vi "Start Build.vi"(0 "Open Directory?":bool, 1 "Build Packge?":bool, 2 "Progres Bar":refnum<vi>, 5 "Feed":T2(ring), 7 "Feed Path":path, 9 "Selected Measurements":T1[](array[typedef]), 11 "error in (no error)":errorcluster, 12 "Package Spec":string[][](array[string])) -> (4 "Status":string[](array[string]), 15 "error out":errorcluster)   [LabVIEW 2021, in "Packager Helpers.lvlib"]
uses:
  Packager Helpers.lvlib
  controls/Build Spec Details.ctl
  <vilib>/AppBuilder/AB_API_Simple/Set Build Specification Version (path).vi
  <vilib>/AppBuilder/AB_API_Simple/Build (path).vi
  Dictionary/Dictionary.lvlib
  <vilib>/AppBuilder/AB_API_Simple/NI_App_Builder_API.lvlib
  Path Functions/Path Functions.lvlib
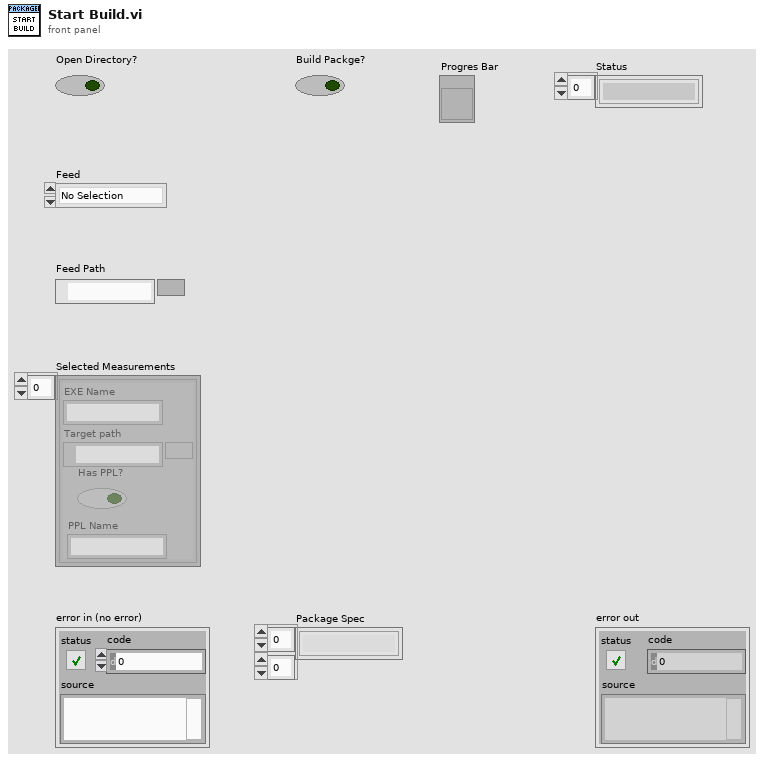
[diagram p1: front panel]
types:
  T1 = typedef "Packager Helpers.lvlib/Build Spec Details.ctl" = cluster{"EXE Name":string, "Target path":path, "Has PPL?":bool, "PPL Name":string}
  T2 = enum32{"No Selection", "CreateFeed", "AddtoFeed"}
  T3 = typedef "NI_App_Builder_API.lvlib/Build Specification Version.ctl" = cluster{"Major":u16, "Minor":u16, "Fix":u16, "Build":u16}
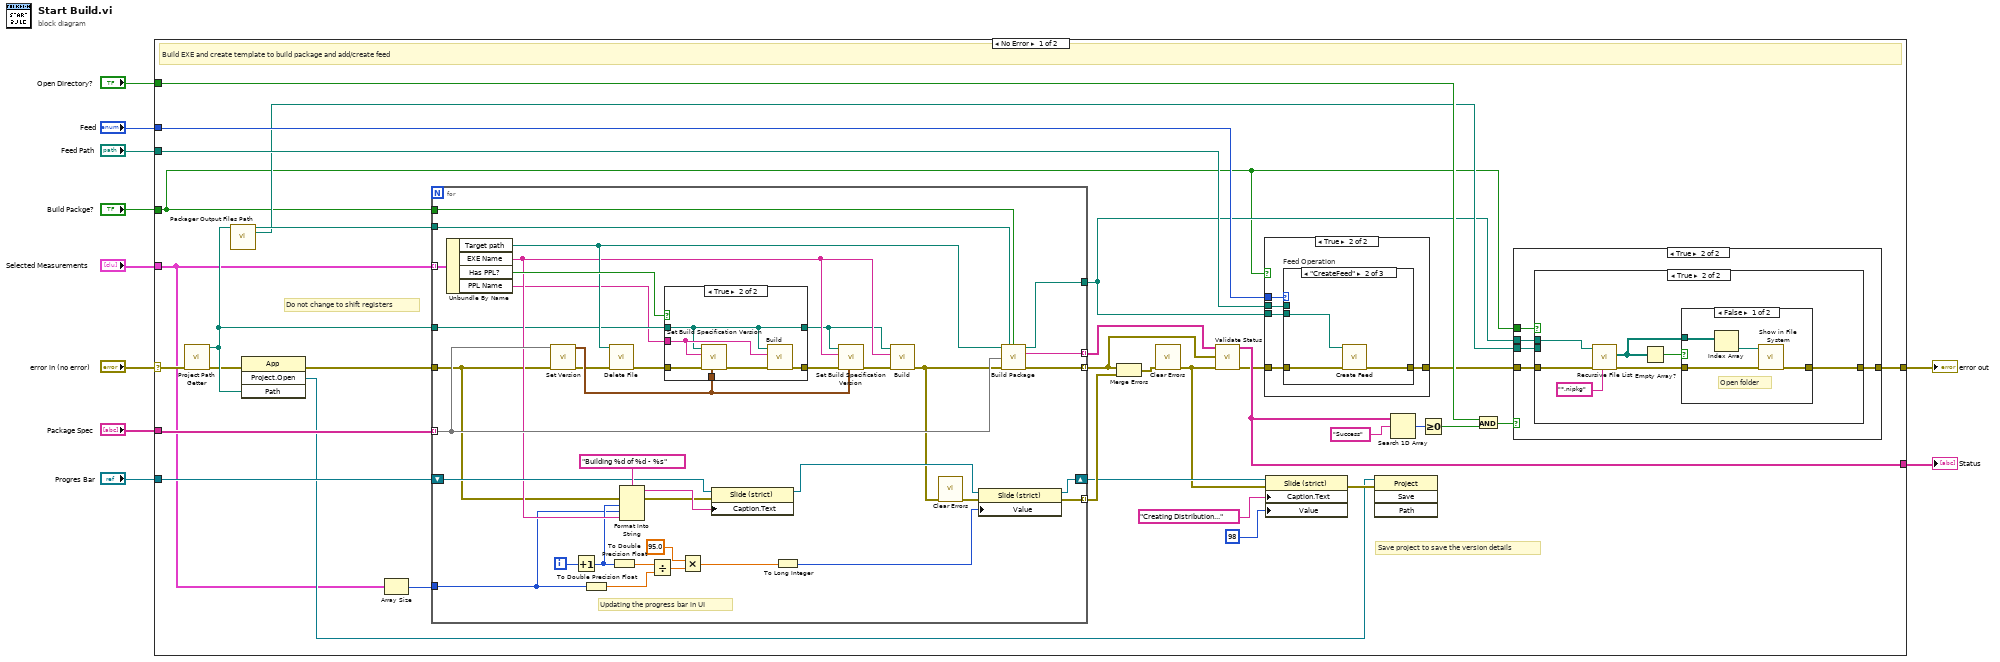
[diagram p0: block diagram]
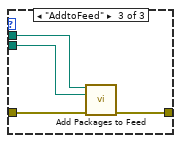
[diagram p4: hidden frame]
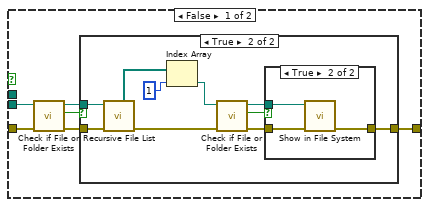
[diagram p7: hidden frame]
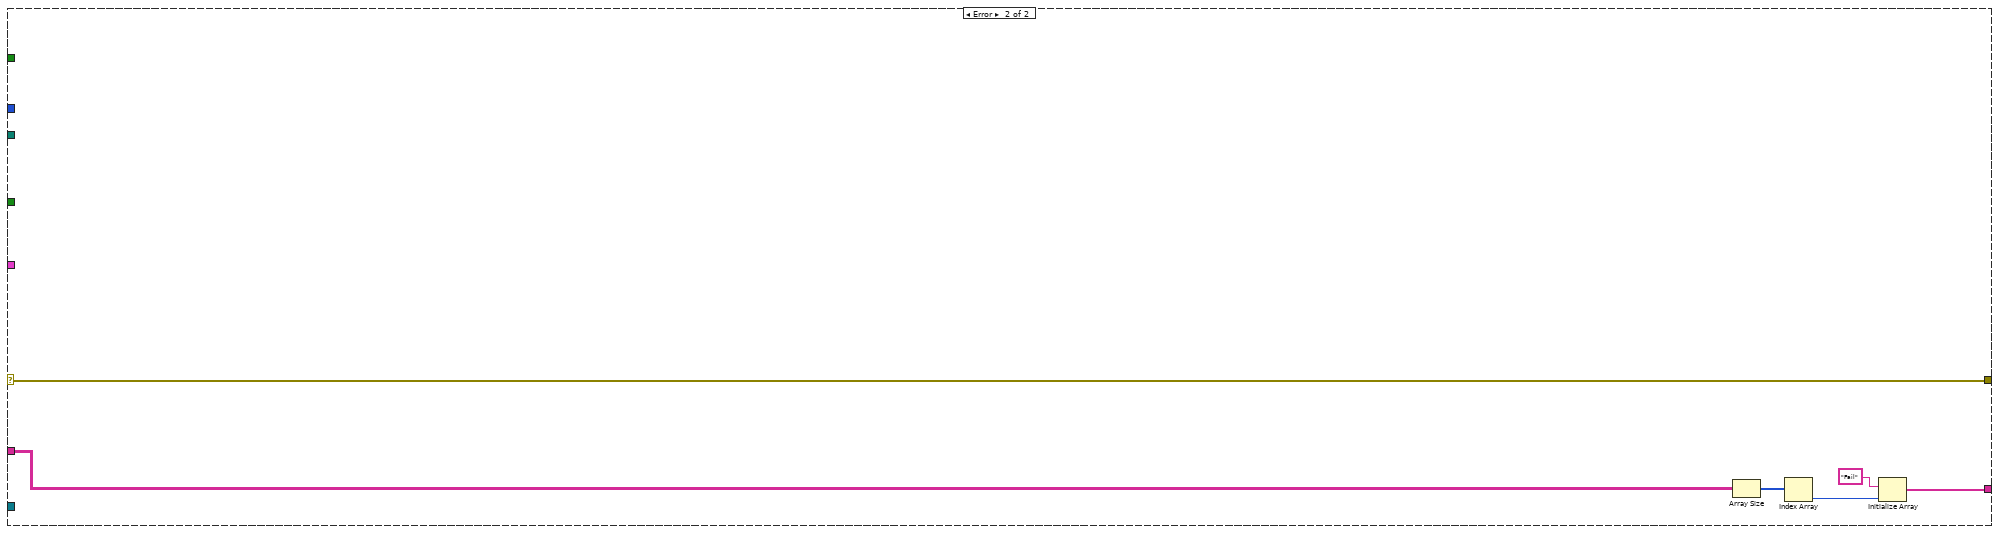
[diagram p11: hidden frame]
diagram:
  n1 = case shown="No Error" "error in (no error)" {
    selector: "error in (no error)" -> [w29 w142]
    tunnel: "Package Spec" -> [w43 w147]
    tunnel: [w37 w144] -> w9
    tunnel: "Progres Bar" -> [w27 _]
    tunnel: "Open Directory?" -> [w33 _]
    tunnel: "Feed" -> [w39 _]
    tunnel: "Feed Path" -> [w38 _]
    tunnel: "Build Packge?" -> [w13 _]
    tunnel: "Selected Measurements" -> [w20 _]
    tunnel: [w14 w142] -> w10
    frame No Error {
      # "Do not change to shift registers"
      # "Save project to save the version details"
      # "Build EXE and create template to build package and add/create feed"
      n2 = call "Project Path Getter.vi"("error in (no error)"=w29) -> ("Path"=w31:path, "error out"=w28:errorcluster)  [unwired: 13 in]
      n3 = call "Packager Output Files Path.vi"("Project Path"=w31) -> ("Package Path"=w32:path, "Build Outputs Path"=w30:path)  [unwired: 13 in]
      n4 = invoke class="App" method="Project.Open"(error in=w28, "Path"=w31) -> (error out=w11:errorcluster, "Project:Open"=w21:refnum<vi>)  [unwired: 2 in, 2 out]
      n5 = Array Size(array=w20) -> (size(s)=w41:i32)
      n6 = for {
        tunnel: w11 -> [w69]
        tunnel: w20 -> [w94] mode=indexing
        tunnel: w13 -> [w84]
        tunnel: w43 -> [w77] mode=indexing
        tunnel: [w93] -> w17
        tunnel: [w62] -> w25 mode=indexing
        tunnel: [w92] -> w42 mode=indexing
        tunnel: w41 -> [w59]
        tunnel: [w81] -> w40 mode=indexing
        shift-right: [w79] -> w24
        shift-left: w27 -> [w90]
        tunnel: w31 -> [w72]
        tunnel: w32 -> [w75]
        i -> [w58]
        # "Updating the progress bar in UI"
        n7 = Unbundle By Name(w94) -> ("Target path"=w76:path, "EXE Name"=w73:string, "Has PPL?"=w78:bool, "PPL Name"=w71:string)
        n8 = call "Set Version.vi"("Package Spec"=w77, "error in (no error)"=w69) -> ("Build Specification Version"=w70:T3, "error out"=w68:errorcluster)  [unwired: 12 in]
        n9 = Increment(x=w58) -> (x+1=w60:i32)
        n10 = To Double Precision Float(number=w59) -> (double precision float=w83:dbl)
        n11 = call "Delete File.vi"("File or Folder Path"=w76, "error in (no error)"=w68) -> ("error out"=w67:errorcluster)  [unwired: 13 in]
        n12 = To Double Precision Float(number=w60) -> (double precision float=w85:dbl)
        n13 = Format Into String(format string="Building %d of %d - %s", error in=w69, w60, w59, w73) -> (resulting string=w89:string, error out=w61:errorcluster)  [unwired: 1 in]
        n14 = Divide(x=w85, y=w83) -> (x/y=w88:dbl)
        n15 = case shown="True" w78 {
          tunnel: w72 -> [w95 w97]
          tunnel: w70 -> [_ w102]
          tunnel: w71 -> [_ w101]
          tunnel: w67 -> [w96 w100]
          tunnel: [w96 w98] -> w66
          tunnel: [w95 w97] -> w65
          frame False {
          }
          frame True {
            n16 = call-poly <vilib>:"Set Build Specification Version.vi"("Build Specification Version"=w102, "error in (no error)"=w100, "Name of build specification"=w101, "Path to project"=w97) -> ("error out"=w99:errorcluster)  [unwired: 7 in]
            n17 = call-poly <vilib>:"Build.vi"("error in (no error)"=w99, "Name of build specification (if empty: build all)"=w101, "Path to project"=w97) -> ("error out"=w98:errorcluster)  [unwired: 7 in, 1 out]
          }
        }
        n18 = Multiply(x=95.0 ("y"), y=w88) -> (x*y=w86:dbl)
        n19 = property class="Slide (strict)"(reference=w90, error in=w61, "Caption.Text"=w89) -> (reference out=w74:refnum<vi>)  [unwired: 1 out]
        n20 = To Long Integer(number=w86) -> (32bit integer=w80:i32)
        n21 = call-poly <vilib>:"Set Build Specification Version.vi"("Build Specification Version"=w70, "error in (no error)"=w66, "Name of build specification"=w73, "Path to project"=w65) -> ("error out"=w64:errorcluster)  [unwired: 7 in]
        n22 = call-poly <vilib>:"Build.vi"("error in (no error)"=w64, "Name of build specification (if empty: build all)"=w73, "Path to project"=w65) -> ("error out"=w63:errorcluster)  [unwired: 7 in, 1 out]
        n23 = call <vilib>:"Clear Errors.vi"("error in (no error)"=w63) -> ("error out"=w82:errorcluster)  [unwired: 5 in, 1 out]
        n24 = property class="Slide (strict)"(reference=w74, error in=w82, "Value"=w80) -> (reference out=w79:refnum<vi>, error out=w81:errorcluster)
        n25 = call "Build Package.vi"("Destination Path"=w76, "Package Path"=w75, "Build Package?"=w84, "Package Spec"=w77, "error in (no error)"=w63) -> ("Package Directory"=w93:path, "Error Message"=w92:string, "error out"=w62:errorcluster)  [unwired: 8 in]
      }
      n26 = Merge Errors(w25, w40) -> (w26:errorcluster)
      n27 = call <vilib>:"Clear Errors.vi"("error in (no error)"=w26) -> ("error out"=w23:errorcluster)  [unwired: 5 in, 1 out]
      n28 = call "Validate Status.vi"("Error Msg[]"=w42, "Error[]"=w25, "error in (no error)"=w23) -> ("Status"=w37:string[], "error out"=w16:errorcluster)  [unwired: 11 in]
      n29 = case shown="True" w13 {
        tunnel: w39 -> [_ w49]
        tunnel: w38 -> [_ w48]
        tunnel: w17 -> [_ w47]
        tunnel: w16 -> [w44 w46]
        tunnel: [w44 w45] -> w15
        frame False {
        }
        frame True {
          n30 = case "Feed Operation" shown="\"CreateFeed\"" w49 {
            tunnel: w48 -> [_ _ w57]
            tunnel: w47 -> [_ w53 w56]
            tunnel: w46 -> [w50 w52 w55]
            tunnel: [w50 w51 w54] -> w45
            frame "No Selection" {
            }
            frame "CreateFeed" {
              n31 = call "Create Feed.vi"("Packages Path"=w53, "error in (no error)"=w52) -> ("error out"=w51:errorcluster)  [unwired: 13 in]
            }
            frame "AddtoFeed" {
              n32 = call "Add Packages to Feed.vi"("Feed Path"=w57, "Packages Path"=w56, "error in (no error)"=w55) -> ("error out"=w54:errorcluster)  [unwired: 12 in]
            }
          }
        }
      }
      n33 = property class="Slide (strict)"(reference=w24, error in=w23, "Caption.Text"="Creating Distribution...", "Value"=98) -> (error out=w22:errorcluster)  [unwired: 1 out]
      n34 = invoke class="Project" method="Save"(reference=w21, error in=w22) -> ()  [unwired: 2 in, 4 out]
      n35 = Search 1D Array(1D array=w37, element="Success") -> (index of element=w35:i32)  [unwired: 1 in]
      n36 = Greater Or Equal To 0?(x=w35) -> (x >= 0?=w34:bool)
      n37 = And(x=w33, y=w34) -> (x .and. y?=w12:bool)
      n38 = case shown="True" w12 {
        tunnel: w17 -> [_ w108]
        tunnel: w30 -> [_ w107]
        tunnel: [w103 w105] -> w14
        tunnel: w15 -> [w103 w106]
        tunnel: w13 -> [_ w104]
        frame False {
        }
        frame True {
          n39 = case shown="True" w104 {
            tunnel: w108 -> [_ w136]
            tunnel: w107 -> [w113 _]
            tunnel: w106 -> [w112 w135]
            tunnel: [w110 w131] -> w105
            frame False {
              n40 = call <vilib>:"Check if File or Folder Exists.vi"("error in (no error)"=w112, "path"=w113) -> ("error out"=w111:errorcluster, "file or folder exists?"=w114:bool, "dup path"=w109:path)  [unwired: 7 in]
              n41 = case shown="True" w114 {
                tunnel: w111 -> [w115 w122]
                tunnel: [w115 w117] -> w110
                tunnel: w109 -> [_ w116]
                frame False {
                }
                frame True {
                  n42 = call <vilib>:"Recursive File List.vi"("error in (no error)"=w122, "Folder Path"=w116) -> ("error out"=w120:errorcluster, "All Folders"=w125:path[])  [unwired: 5 in, 3 out]
                  n43 = Index Array(array=w125, index=1) -> (element=w124:path)
                  n44 = call <vilib>:"Check if File or Folder Exists.vi"("error in (no error)"=w120, "path"=w124) -> ("error out"=w123:errorcluster, "file or folder exists?"=w119:bool, "dup path"=w118:path)  [unwired: 7 in]
                  n45 = case shown="True" w119 {
                    tunnel: w123 -> [w126 w128]
                    tunnel: w118 -> [_ w129]
                    tunnel: [w126 w127] -> w117
                    frame False {
                    }
                    frame True {
                      n46 = call <vilib>:"Show in File System.vi"("error in (no error)"=w128, "file or directory path"=w129) -> ("error out"=w127:errorcluster)  [unwired: 9 in]
                    }
                  }
                }
              }
            }
            frame True {
              n47 = call <vilib>:"Recursive File List.vi"("pattern"="*.nipkg", "error in (no error)"=w135, "Folder Path"=w136) -> ("error out"=w132:errorcluster, "All Files in Dir"=w134:path[])  [unwired: 4 in, 3 out]
              n48 = Empty Array?(array=w134) -> (empty?=w133:bool)
              n49 = case shown="False" w133 {
                tunnel: w132 -> [w138 w141]
                tunnel: w134 -> [w140 _]
                tunnel: [w137 w141] -> w131
                frame False {
                  # "Open folder"
                  n50 = Index Array(array=w140) -> (element=w139:path)  [unwired: 1 in]
                  n51 = call <vilib>:"Show in File System.vi"("error in (no error)"=w138, "file or directory path"=w139) -> ("error out"=w137:errorcluster)  [unwired: 9 in]
                }
                frame True {
                }
              }
            }
          }
        }
      }
    }
    frame Error {
      n52 = Array Size(array=w147) -> (size(s)=w146:i32[])
      n53 = Index Array(array=w146) -> (element=w145:i32)  [unwired: 1 in]
      n54 = Initialize Array("Fail", w145) -> (w144:string[])
    }
  }
  "error out" <- w10
  "Status" <- w9
